vi "saveViAndLib.vi"(8 "error in (no error)":errorcluster, 10 "arrayOfVi":path[](array[path]), 11 "libRefIn":refnum<vi>) -> (0 "error out":errorcluster, 3 "libRefOut":refnum<vi>)   [LabVIEW 2018]
doc: "Save the update of Vi and LabVIEW library."
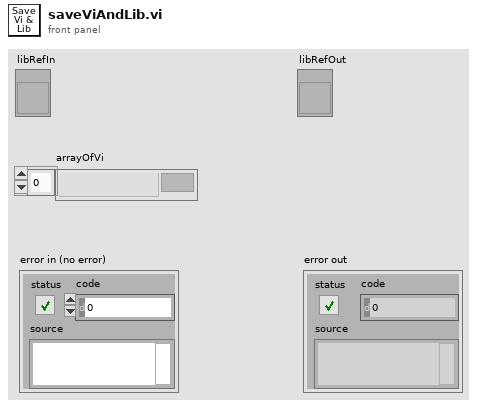
[diagram p1: front panel]
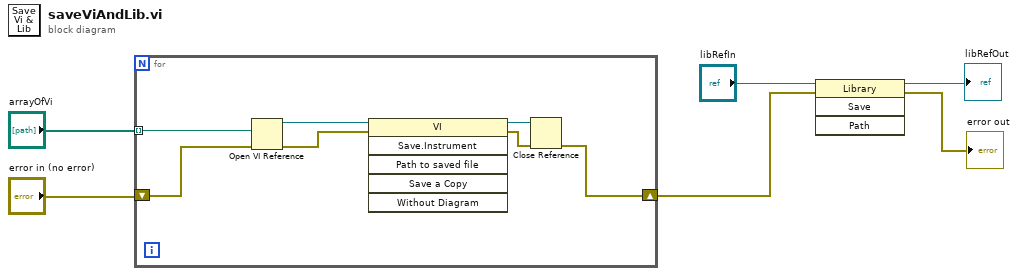
[diagram p0: block diagram]
diagram:
  n1 = for {
    shift-right: [w13] -> w3
    shift-left: "error in (no error)" -> [w8]
    tunnel: "arrayOfVi" -> [w7] mode=indexing
    n2 = Open VI Reference(vi path=w7, error in (no error)=w8) -> (vi reference=w9:refnum<vi>, error out=w10:errorcluster)  [unwired: 4 in]
    n3 = invoke class="VI" method="Save.Instrument"(reference=w9, error in=w10) -> (reference out=w12:refnum<vi>, error out=w11:errorcluster)  [unwired: 4 in, 4 out]
    n4 = Close Reference(reference=w12, error in (no error)=w11) -> (error out=w13:errorcluster)
  }
  n5 = invoke class="Library" method="Save"(reference="libRefIn", error in=w3) -> (reference out=→"libRefOut":refnum<vi>, error out=→"error out":errorcluster)  [unwired: 2 in, 2 out]
